vi "Rendering - Number Format.vi"(5 "format string":string, 6 "Is Lower Coefficient?":bool, 7 "Is Higher Coefficient?":bool, 11 "Coefficient":dbl) -> (3 "String Coefficient":string)   [LabVIEW 2023]
doc: "Format number for rendering in a picture control."
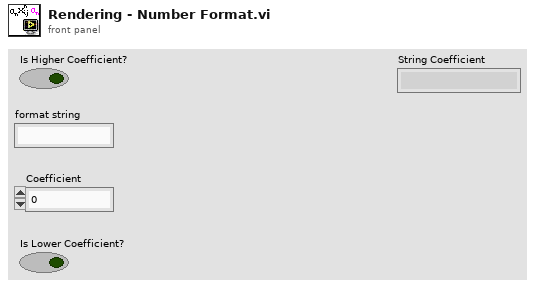
[diagram p1: front panel]
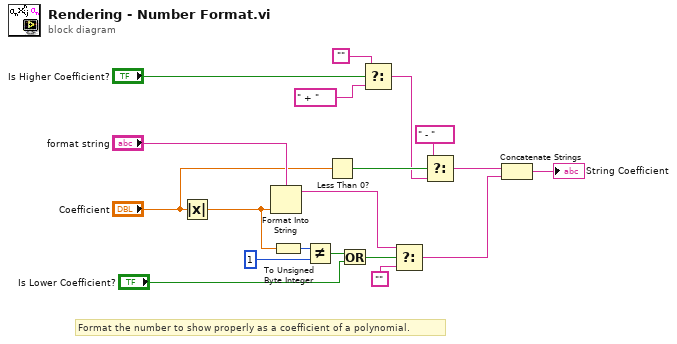
[diagram p0: block diagram]
diagram:
  # "Format the number to show properly as a coefficient of a polynomial."
  n1 = Absolute Value(x="Coefficient") -> (abs(x)=w4:dbl)
  n2 = Format Into String(format string="format string", w4) -> (resulting string=w6:string)  [unwired: 2 in, 1 out]
  n3 = To Unsigned Byte Integer(number=w4) -> (unsigned 8bit integer=w1:u8)
  n4 = Not Equal?(x=w1, y=u8 1) -> (x != y?=w8:bool)
  n5 = Less Than 0?(x="Coefficient") -> (x < 0?=w18:bool)
  n6 = Or(x=w8, y="Is Lower Coefficient?") -> (x .or. y?=w3:bool)
  n7 = Select(t="", s="Is Higher Coefficient?", f=" + " ("string")) -> (s? t:f=w12:string)
  n8 = Select(t=w6, s=w3, f="") -> (s? t:f=w5:string)
  n9 = Select(t=" - " ("string"), s=w18, f=w12) -> (s? t:f=w11:string)
  n10 = Concatenate Strings(w11, w5) -> (→"String Coefficient":string)
